vi "Immediate Children.vi"(8 "error in":errorcluster, 10 "Object":refnum<class>) -> (0 "error out":errorcluster, 2 "Immediate Children Paths":path[](array[path]))   [LabVIEW 2021, in "_Shared.lvlib"]
uses:
  _Shared.lvlib
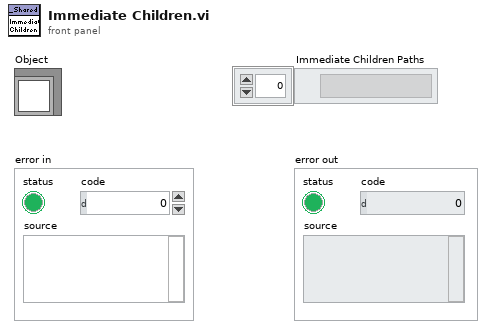
[diagram p1: front panel]
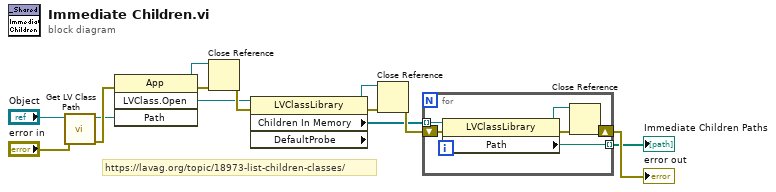
[diagram p0: block diagram]
diagram:
  # "https://lavag.org/topic/18973-list-children-classes/"
  n1 = call <vilib>:"Get LV Class Path.vi"("error in (no error)"="error in", "object"="Object") -> ("error out"=w8:errorcluster, "class path"=w7:path)  [unwired: 8 in]
  n2 = invoke class="App" method="LVClass.Open"(error in=w8, "Path"=w7) -> (reference out=w14:refnum<vi>, error out=w13:errorcluster, "LVClass.Open"=w11:refnum<vi>)  [unwired: 2 in, 1 out]
  n3 = Close Reference(reference=w14, error in (no error)=w13) -> (error out=w12:errorcluster)
  n4 = property class="LVClassLibrary" props=["Children In Memory", "DefaultProbe"](reference=w11, error in=w12) -> (reference out=w9:refnum<vi>, error out=w10:errorcluster, "Children In Memory"=w5:refnum<vi>[])  [unwired: 1 out]
  n5 = Close Reference(reference=w9, error in (no error)=w10) -> (error out=w6:errorcluster)
  n6 = for {
    tunnel: w5 -> [w19] mode=indexing
    shift-right: [w16] -> w2
    shift-left: w6 -> [w20]
    tunnel: [w15] -> w1 mode=indexing
    n7 = property class="LVClassLibrary"(reference=w19, error in=w20) -> (reference out=w17:refnum<vi>, error out=w18:errorcluster, "Path"=w15:path)
    n8 = Close Reference(reference=w17, error in (no error)=w18) -> (error out=w16:errorcluster)
  }
  "error out" <- w2
  "Immediate Children Paths" <- w1
